vi "6812B_AC_Output.vi"() -> ()   [LabVIEW 2019]
doc: "Shows how to generate a standard output."
uses:
  <instrlib>/Agilent 681x Series/Agilent 681x Series.lvlib
panel:
  in  "Pulse Characteristic Value (%)":dbl=50.0 format="%#.4g"
  in  "Pulse Characteristic (0: Duty Cycle)":u16(ring) items=["Duty Cycle", "Pulse Width"]
  in  "Period (s)":dbl=0.03333 format="%#.4g"
  in  "Trigger Delay (s)":dbl format="%#.5g"
  in  "Pulse Count":dbl=1.0 format="%#.4g"
  in  "Voltage Mode (0: Fix)":u16(ring) items=["Fixed", "Step", "Pulse", "List"]
  in  "Triggered Voltage Amplitude (V)":dbl=1.0 format="%#.4g"
  in  "Parar o programa":bool
  in  "Peak Current Limit (13 A)":dbl=13.0 format="%#.4g"
  in  "RMS Current Limit (1 A)":dbl=1.0 format="%#.4g"
  in  "Voltage Amplitude (1.0 V)":dbl=1.0 format="%#.4g"
  in  "Output Frequency (60 Hz)":dbl=60.0 format="%#.4g"
  in  "Output Waveform Type (0: Sinusoid)":u16(ring) items=["Sinusoid", "Square", "Clipped Sinusoid", "User Specified"]
  in  "Serial Configuration":T1={"Baud Rate"=9600, "Parity"=0, "Data Bits"=8} {"Data Bits" items=["7"=7, "8"=8]; "Parity" items=["None", "Odd", "Even", "Mark", "Space"]; "Baud Rate" items=["300"=300, "600"=600, "1200"=1200, "2400"=2400, "4800"=4800, "9600"=9600]}
  in  "VISA resource name":refnum<visa-resource-name>
  # "(c) 2008-2021 National Instruments Corp.  ALL RIGHTS RESERVED."
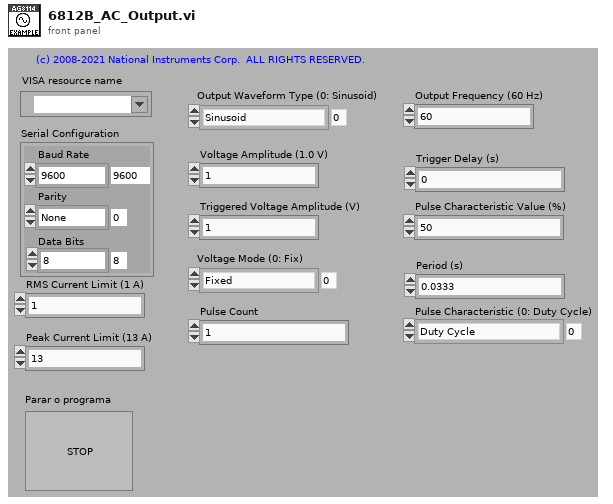
[diagram p1: front panel]
types:
  T1 = cluster{"Baud Rate":u32, "Parity":u16, "Data Bits":u16}
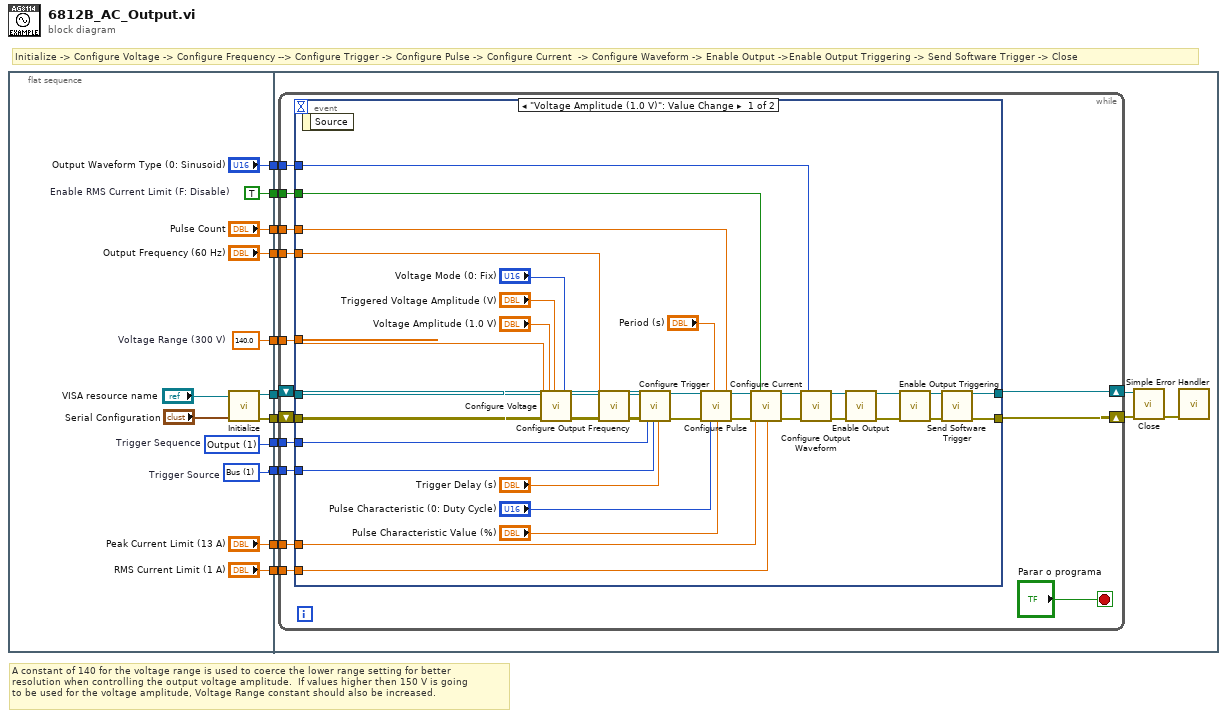
[diagram p0: block diagram]
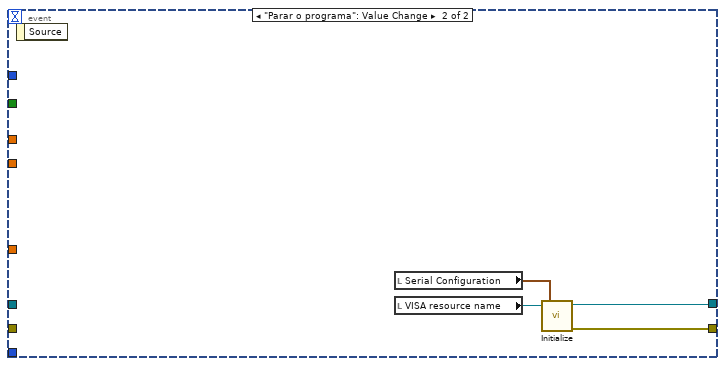
[diagram p2: hidden frame]
diagram:
  # "Initialize -> Configure Voltage -> Configure Frequency --> Configure Trigger -> Configure Pulse -> Configure Current  -> Configure Waveform -> Enable Output ->Enable Output Triggering -> Send Software Trigger -> Close"
  # "A constant of 140 for the voltage range is used to coerce the lower range setting for better\nresolution when controlling the output voltage amplitude.  If values higher then 150 V is going\nto be used for the voltage amplitude, Voltage Range constant should also be increased."
  n1 = flat-sequence {
    tunnel: [w24] -> w11
    tunnel: [w23] -> w10
    tunnel: ["Output Waveform Type (0: Sinusoid)"] -> w9
    tunnel: [w21] -> w8
    tunnel: [w20] -> w7
    tunnel: ["Output Frequency (60 Hz)"] -> w6
    tunnel: ["RMS Current Limit (1 A)"] -> w5
    tunnel: ["Peak Current Limit (13 A)"] -> w4
    tunnel: ["Pulse Count"] -> w3
    tunnel: [w13] -> w2
    tunnel: [w12] -> w1
    tunnel: w11 -> [w35]
    tunnel: w10 -> [w34]
    tunnel: w9 -> [w33]
    tunnel: w8 -> [w32]
    tunnel: w7 -> [w31]
    tunnel: w6 -> [w30]
    tunnel: w5 -> [w29]
    tunnel: w4 -> [w28]
    tunnel: w3 -> [w27]
    tunnel: w2 -> [w26]
    tunnel: w1 -> [w25]
    frame #0 {
      w12 = 1 items=["Immediate", "Bus", "External", "Phase", "Trigger Out"]  # Trigger Source
      w13 = 1 items=["Output"=1, "Synchronous Source"=2, "Measurement"=3]  # Trigger Sequence
      w20 = TRUE  # Enable RMS Current Limit (F: Disable)
      w21 = 140.0  # Voltage Range (300 V)
      n2 = call <instrlib>:"Initialize.vi"("Serial Configuration"="Serial Configuration", "VISA resource name"="VISA resource name") -> ("error out"=w23:errorcluster, "VISA resource name out"=w24:refnum<visa-resource-name>)  [unwired: 8 in]
    }
    frame #1 {
      n3 = while {
        tunnel: w33 -> [w48]
        tunnel: w32 -> [w47]
        tunnel: w31 -> [w46]
        tunnel: w30 -> [w45]
        tunnel: w29 -> [w44]
        tunnel: w28 -> [w43]
        shift-right: [w52] -> w37
        shift-left: w35 -> [w50]
        shift-right: [w51] -> w36
        shift-left: w34 -> [w49]
        tunnel: w27 -> [w41]
        tunnel: w26 -> [w40]
        tunnel: w25 -> [w39]
        stop <- "Parar o programa" stop-if-true
        n4 = event shown="[0] \"Voltage Amplitude (1.0 V)\": Value Change" {
          selector: _ -> [_ _]
          dyn-events: _ -> [_ _]
          timeout: _ -> [_ _]
          tunnel: w50 -> [w88 _]
          tunnel: w49 -> [w87 _]
          tunnel: w48 -> [w86 _]
          tunnel: w47 -> [w85 _]
          tunnel: w46 -> [w82 _]
          tunnel: [w62 w92] -> w51
          tunnel: [w63 w91] -> w52
          tunnel: w45 -> [w76 _]
          tunnel: w44 -> [w81 _]
          tunnel: w43 -> [w80 _]
          tunnel: w41 -> [w61 _]
          tunnel: w40 -> [w56 _]
          tunnel: w39 -> [w55 _]
          event "Voltage Amplitude (1.0 V)": Value Change {
            n5 = event-data() -> ()  [unwired: 1 in, 1 out]
            n6 = call <instrlib>:"Configure Voltage.vi"("VISA resource name"=w88, "Triggered Voltage Amplitude (1.0 V)"="Triggered Voltage Amplitude (V)", "Voltage Range (300 V)"=w85, "Voltage Amplitude (1.0 V)"="Voltage Amplitude (1.0 V)", "Voltage Mode (0: Fix)"="Voltage Mode (0: Fix)", "error in (no error)"=w87) -> ("VISA resource name out"=w78:refnum<visa-resource-name>, "error out"=w77:errorcluster)  [unwired: 8 in]
            n7 = call <instrlib>:"Configure Output Frequency.vi"("VISA resource name"=w78, "Output Frequency (60 Hz)"=w76, "error in (no error)"=w77) -> ("VISA resource name out"=w75:refnum<visa-resource-name>, "error out"=w74:errorcluster)  [unwired: 11 in]
            n8 = call <instrlib>:"Configure Trigger.vi"("VISA resource name"=w75, "Trigger Sequence (1: Output 1)"=w56, "Trigger Source (0: Immediate)"=w55, "error in (no error)"=w74, "Trigger Delay (0 s)"="Trigger Delay (s)") -> ("VISA resource name out"=w73:refnum<visa-resource-name>, "error out"=w72:errorcluster)  [unwired: 9 in]
            n9 = call <instrlib>:"Configure Pulse.vi"("VISA resource name"=w73, "Pulse Count (1)"=w61, "Period (0.0333 s)"="Period (s)", "error in (no error)"=w72, "Pulse Characteristic (0: Duty Cycle)"="Pulse Characteristic (0: Duty Cycle)", "Pulse Characteristic Value (50)"="Pulse Characteristic Value (%)") -> ("VISA resource name out"=w71:refnum<visa-resource-name>, "error out"=w70:errorcluster)  [unwired: 8 in]
            n10 = call <instrlib>:"Configure Current.vi"("VISA resource name"=w71, "Enable RMS Current Limit (F: Disable)"=w82, "RMS Current Limit (1 A)"=w81, "error in (no error)"=w70, "Peak Current Limit (13 A)"=w80) -> ("VISA resource name out"=w69:refnum<visa-resource-name>, "error out"=w68:errorcluster)  [unwired: 9 in]
            n11 = call <instrlib>:"Configure Output Waveform.vi"("VISA resource name"=w69, "Output Waveform Type (0: Sinusoid)"=w86, "error in (no error)"=w68) -> ("VISA resource name out"=w83:refnum<visa-resource-name>, "error out"=w84:errorcluster)  [unwired: 11 in]
            n12 = call <instrlib>:"Enable Output.vi"("VISA resource name"=w83, "error in (no error)"=w84) -> ("VISA resource name out"=w65:refnum<visa-resource-name>, "error out"=w64:errorcluster)  [unwired: 12 in]
            n13 = call <instrlib>:"Enable Output Triggering.vi"("VISA resource name"=w65, "error in (no error)"=w64) -> ("VISA resource name out"=w66:refnum<visa-resource-name>, "error out"=w67:errorcluster)  [unwired: 12 in]
            n14 = call <instrlib>:"Send Software Trigger.vi"("VISA resource name"=w66, "error in (no error)"=w67) -> ("VISA resource name out"=w63:refnum<visa-resource-name>, "error out"=w62:errorcluster)  [unwired: 12 in]
          }
          event "Parar o programa": Value Change {
            n15 = event-data() -> ()  [unwired: 1 in, 1 out]
            n16 = local read "Serial Configuration"() -> (w89:T1)
            n17 = local read "VISA resource name"() -> (w90:refnum<visa-resource-name>)
            n18 = call <instrlib>:"Initialize.vi"("Serial Configuration"=w89, "VISA resource name"=w90) -> ("error out"=w92:errorcluster, "VISA resource name out"=w91:refnum<visa-resource-name>)  [unwired: 8 in]
          }
        }
      }
      n19 = call <instrlib>:"Close.vi"("error in (no error)"=w36, "VISA resource name"=w37) -> ("error out"=w38:errorcluster)  [unwired: 9 in]
      n20 = call <vilib>:"Simple Error Handler.vi"("error in (no error)"=w38) -> ()  [unwired: 4 in, 5 out]
    }
  }
